vi "GetTDMSLogFilePath.vi"(7 "Set? (F)":bool, 11 ".tst file":path) -> (3 "TDMS Log File Path":path)   [LabVIEW 2018, in "Test.lvclass"]
doc: "Functional Global Variable that holds an array of modules in use."
uses:
  Test.lvclass
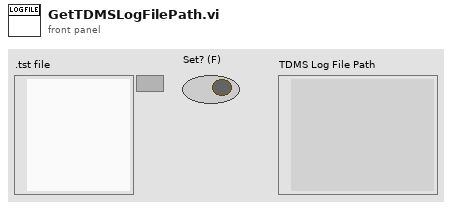
[diagram p1: front panel]
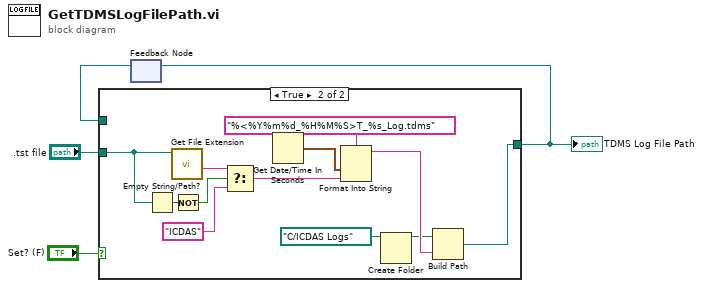
[diagram p0: block diagram]
diagram:
  n1 = feedback #1() -> (w3:path)  [unwired: 1 in]
  n2 = case shown="True" "Set? (F)" {
    tunnel: [w5 w8] -> w1
    tunnel: ".tst file" -> [_ w16]
    tunnel: w3 -> [w5 _]
    frame False {
    }
    frame True {
      n3 = Empty String/Path?(string/path=w16) -> (empty?=w15:bool)
      n4 = call <vilib>:"Get File Extension.vi"("file"=w16) -> ("filename without extension"=w17:string)  [unwired: 6 in, 4 out]
      n5 = Not(x=w15) -> (.not. x?=w14:bool)
      n6 = Select(t=w17, s=w14, f="ICDAS") -> (s? t:f=w6:string)
      n7 = Get Date/Time In Seconds() -> (seconds since 1Jan1904=w7:timestamp)
      n8 = Format Into String(format string="%<%Y%m%d_%H%M%S>T_%s_Log.tdms", w7, w6) -> (resulting string=w10:string)  [unwired: 2 in, 1 out]
      n9 = Create Folder(path (use dialog)=path "C:/ICDAS Logs") -> (created path=w9:path)  [unwired: 2 in, 2 out]
      n10 = Build Path(base path=w9, name or relative path=w10) -> (appended path=w8:path)
    }
  }
  "TDMS Log File Path" <- w1
  n11 = feedback-in #1(w1) -> ()
